vi "Is Post Step Runtime Error.vi"(11 "error in":errorcluster) -> (4 "Is Post Step Runtime Error":bool, 15 "error out":errorcluster)   [LabVIEW 2023, in "RFCalAndFixtureCharact.Common.lvlib"]
uses:
  RFCalAndFixtureCharact.Common.lvlib
  Global Post Step Runtime Error ID.vi
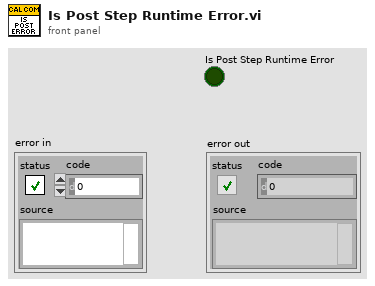
[diagram p1: front panel]
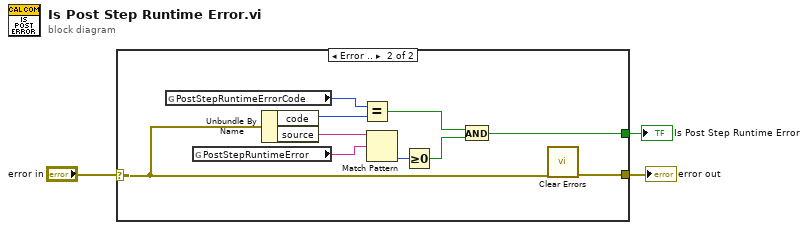
[diagram p0: block diagram]
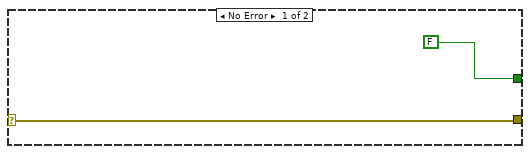
[diagram p2: hidden frame]
diagram:
  n1 = case shown="Error .." "error in" {
    selector: "error in" -> [w4 w11]
    tunnel: [FALSE w10] -> w3
    tunnel: [w4 w12] -> w2
    frame No Error {
    }
    frame Error {
      n2 = global read "Global Post Step Runtime Error ID.vi" "PostStepRuntimeErrorCode"() -> (w13:i32)
      n3 = global read "Global Post Step Runtime Error ID.vi" "PostStepRuntimeError"() -> (w8:string)
      n4 = Unbundle By Name(w11) -> ("code"=w15:i32, "source"=w9:string)
      n5 = Equal?(x=w13, y=w15) -> (x = y?=w14:bool)
      n6 = Match Pattern(string=w9, regular expression=w8) -> (offset past match=w7:i32)  [unwired: 1 in, 3 out]
      n7 = Greater Or Equal To 0?(x=w7) -> (x >= 0?=w6:bool)
      n8 = And(x=w14, y=w6) -> (x .and. y?=w10:bool)
      n9 = call <vilib>:"Clear Errors.vi"("error in (no error)"=w11) -> ("error out"=w12:errorcluster)  [unwired: 5 in, 1 out]
    }
  }
  "Is Post Step Runtime Error" <- w3
  "error out" <- w2
